vi "FilterAirmarGPS.vi"(9 "Queue timeout (ms)":i32=200, 10 "NotifierReff":T1, 11 "AirmarGPS-Compass Queue Cluster":T2) -> ()   [LabVIEW 2013]
doc: "Performs and filtering that we want (default is no filtering) and writes the data to the notifier. If no data is in the queue this VI times out after 'Queue timeout (ms)' has passed and nothing is written to the notifier.\n\nEric Schneider, March 2014"
uses:
  Data/TypeDefs/GPS-Compass Queue Cluster.ctl
  Data/TypeDefs/UTM Location.ctl
  Data/TypeDefs/Notifiers.ctl
  Data/TypeDefs/Sail Set Suggestions.ctl
  Data/TypeDefs/Rudder Set Suggestions.ctl
  Data/TypeDefs/OverrideInformation.ctl
  Data/TypeDefs/OverrideMode.ctl
  Data/TypeDefs/MotorSetup.ctl
  Data/TypeDefs/DynamixelSetupInfo.ctl
  Data/TypeDefs/AirmarStatus.ctl
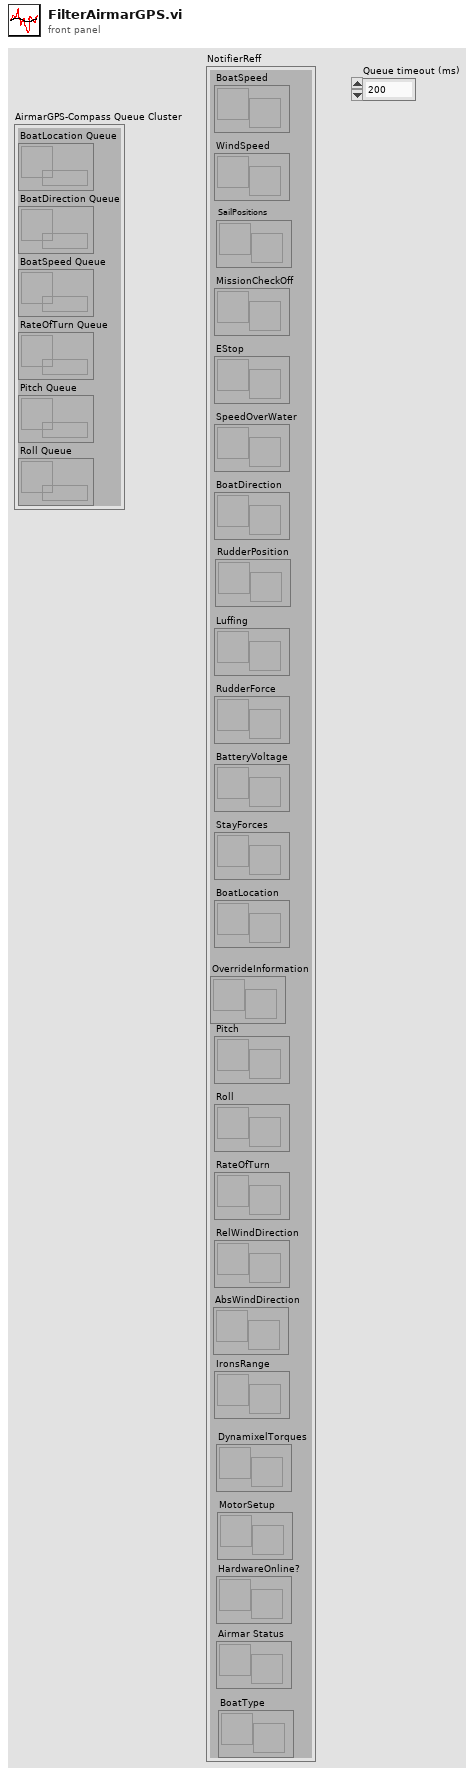
[diagram p1: front panel]
types:
  T1 = typedef "Notifiers.ctl" = cluster{"BoatSpeed":refnum<notifier>, "WindSpeed":refnum<notifier>, "MissionCheckOff":refnum<notifier>, "EStop":refnum<notifier>, "SpeedOverWater":refnum<notifier>, "BoatDirection":refnum<notifier>, "Luffing":refnum<notifier>, "RudderForce":refnum<notifier>, "BatteryVoltage":refnum<notifier>, "StayForces":refnum<notifier>, "BoatLocation":refnum<notifier>, "Pitch":refnum<notifier>, "Roll":refnum<notifier>, "RateOfTurn":refnum<notifier>, "RelWindDirection":refnum<notifier>, "SailPositions":refnum<notifier>, "RudderPosition":refnum<notifier>, "IronsRange":refnum<notifier>, "AbsWindDirection":refnum<notifier>, "OverrideInformation":refnum<notifier>, "DynamixelTorques":refnum<notifier>, "HardwareOnline?":refnum<notifier>, "MotorSetup":refnum<notifier>, "Airmar Status":refnum<notifier>, "BoatType":refnum<notifier>}
  T2 = typedef "GPS-Compass Queue Cluster.ctl" = cluster{"BoatLocation Queue":refnum<queue>, "BoatDirection Queue":refnum<queue>, "BoatSpeed Queue":refnum<queue>, "RateOfTurn Queue":refnum<queue>, "Pitch Queue":refnum<queue>, "Roll Queue":refnum<queue>}
  T3 = typedef "UTM Location.ctl" = cluster{"UTM Zone":dbl, "Hemisphere":enum16{"North", "South"}, "East":dbl, "North":dbl}
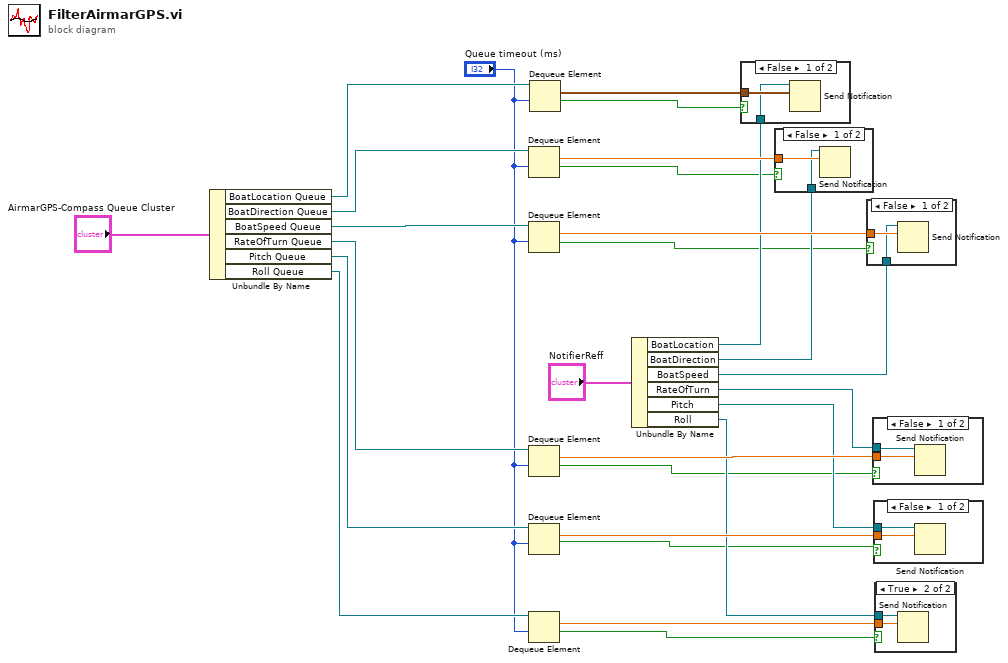
[diagram p0: block diagram]
diagram:
  n1 = Unbundle By Name("AirmarGPS-Compass Queue Cluster") -> ("BoatLocation Queue"=w26:refnum<queue>, "BoatDirection Queue"=w25:refnum<queue>, "BoatSpeed Queue"=w24:refnum<queue>, "RateOfTurn Queue"=w23:refnum<queue>, "Pitch Queue"=w22:refnum<queue>, "Roll Queue"=w21:refnum<queue>)
  n2 = Dequeue Element(queue=w25, timeout in ms (-1)="Queue timeout (ms)") -> (element=w19:dbl, timed out?=w5:bool)  [unwired: 1 in, 2 out]
  n3 = Dequeue Element(queue=w24, timeout in ms (-1)="Queue timeout (ms)") -> (element=w17:dbl, timed out?=w4:bool)  [unwired: 1 in, 2 out]
  n4 = Dequeue Element(queue=w23, timeout in ms (-1)="Queue timeout (ms)") -> (element=w18:dbl, timed out?=w3:bool)  [unwired: 1 in, 2 out]
  n5 = Dequeue Element(queue=w22, timeout in ms (-1)="Queue timeout (ms)") -> (element=w16:dbl, timed out?=w2:bool)  [unwired: 1 in, 2 out]
  n6 = Dequeue Element(queue=w21, timeout in ms (-1)="Queue timeout (ms)") -> (element=w15:dbl, timed out?=w1:bool)  [unwired: 1 in, 2 out]
  n7 = Dequeue Element(queue=w26, timeout in ms (-1)="Queue timeout (ms)") -> (element=w20:T3, timed out?=w6:bool)  [unwired: 1 in, 2 out]
  n8 = Unbundle By Name("NotifierReff") -> ("BoatLocation"=w13:refnum<notifier>, "BoatDirection"=w12:refnum<notifier>, "BoatSpeed"=w11:refnum<notifier>, "RateOfTurn"=w10:refnum<notifier>, "Pitch"=w9:refnum<notifier>, "Roll"=w8:refnum<notifier>)
  n9 = case shown="False" w6 {
    tunnel: w20 -> [w29 _]
    tunnel: w13 -> [w28 _]
    frame False {
      n10 = Send Notification(notification=w29, notifier=w28) -> ()  [unwired: 1 in, 2 out]
    }
    frame True {
    }
  }
  n11 = case shown="False" w5 {
    tunnel: w19 -> [w31 _]
    tunnel: w12 -> [w30 _]
    frame False {
      n12 = Send Notification(notification=w31, notifier=w30) -> ()  [unwired: 1 in, 2 out]
    }
    frame True {
    }
  }
  n13 = case shown="False" w4 {
    tunnel: w17 -> [w33 _]
    tunnel: w11 -> [w32 _]
    frame False {
      n14 = Send Notification(notification=w33, notifier=w32) -> ()  [unwired: 1 in, 2 out]
    }
    frame True {
    }
  }
  n15 = case shown="False" w3 {
    tunnel: w18 -> [w35 _]
    tunnel: w10 -> [w34 _]
    frame False {
      n16 = Send Notification(notification=w35, notifier=w34) -> ()  [unwired: 1 in, 2 out]
    }
    frame True {
    }
  }
  n17 = case shown="False" w2 {
    tunnel: w16 -> [w37 _]
    tunnel: w9 -> [w36 _]
    frame False {
      n18 = Send Notification(notification=w37, notifier=w36) -> ()  [unwired: 1 in, 2 out]
    }
    frame True {
    }
  }
  n19 = case shown="True" w1 {
    tunnel: w15 -> [_ w39]
    tunnel: w8 -> [_ w38]
    frame False {
    }
    frame True {
      n20 = Send Notification(notification=w39, notifier=w38) -> ()  [unwired: 1 in, 2 out]
    }
  }
